vi "CRYMain.vi"() -> ()   [LabVIEW 2013]
uses:
  CRYMainGlobal.vi
  CRYProject/CRYProject Editor Global.vi
  CRYSystem/Task Sequence/CRYProject Run Control Global.vi
  CRYSystem/Data/CRYData & result stacks global.vi
  CRYCurveLibrary/Global/CRYCurve Library Global.vi
panel:
  in  "Tested:":string caption="己测:"
  in  "Curve Library":bool
  in  "OneSetup":bool
  in  "OneCalMic":bool
  in  "OneSelfTest":bool
  in  "Seq Continue":bool
  in  "Wave Lib":bool
  in  "TF Lib":bool
  in  "Value Lib":bool
  in  "SetCalibration":bool
  in  "SetSoundCard":bool
  out "Elapsed":string="00.00"
  in  "Pause":bool
  in  "S/N:":string caption="序号:"
  in  "Lot:":string caption="品名:"
  in  "Manual":bool
  in  "About":bool
  in  "Company Site":bool
  in  "RTA":bool
  in  "Spectral":bool
  in  "Oscillo":bool
  in  "MultiMeter":bool
  in  "SignalGen":bool
  in  "Document":bool
  in  "Data View":bool
  in  "Step Setup":bool
  in  "Curve Lib":bool
  in  "Project":bool
  in  "Pre Window:State":T1(ring)
  in  "DockCommand":string
  out "DockInsert":i32
  in  "Redo":bool
  in  "Continue":bool
  in  "Start":bool
  in  "AddStep":bool
  out "Seq cont border":bool
  in  "stop":bool
  in  "Calibration setup":string
  in  "Hardware setup":string
  out "no key":bool
  out "Key Val":string
  in  "Seq running":bool
  out "Verdict":bool
  out "Margin":string="0.0"
  out "Category Name":string
  in  "StateName":string
  out "State":u8(slide)=49 scale=0.0..100.0
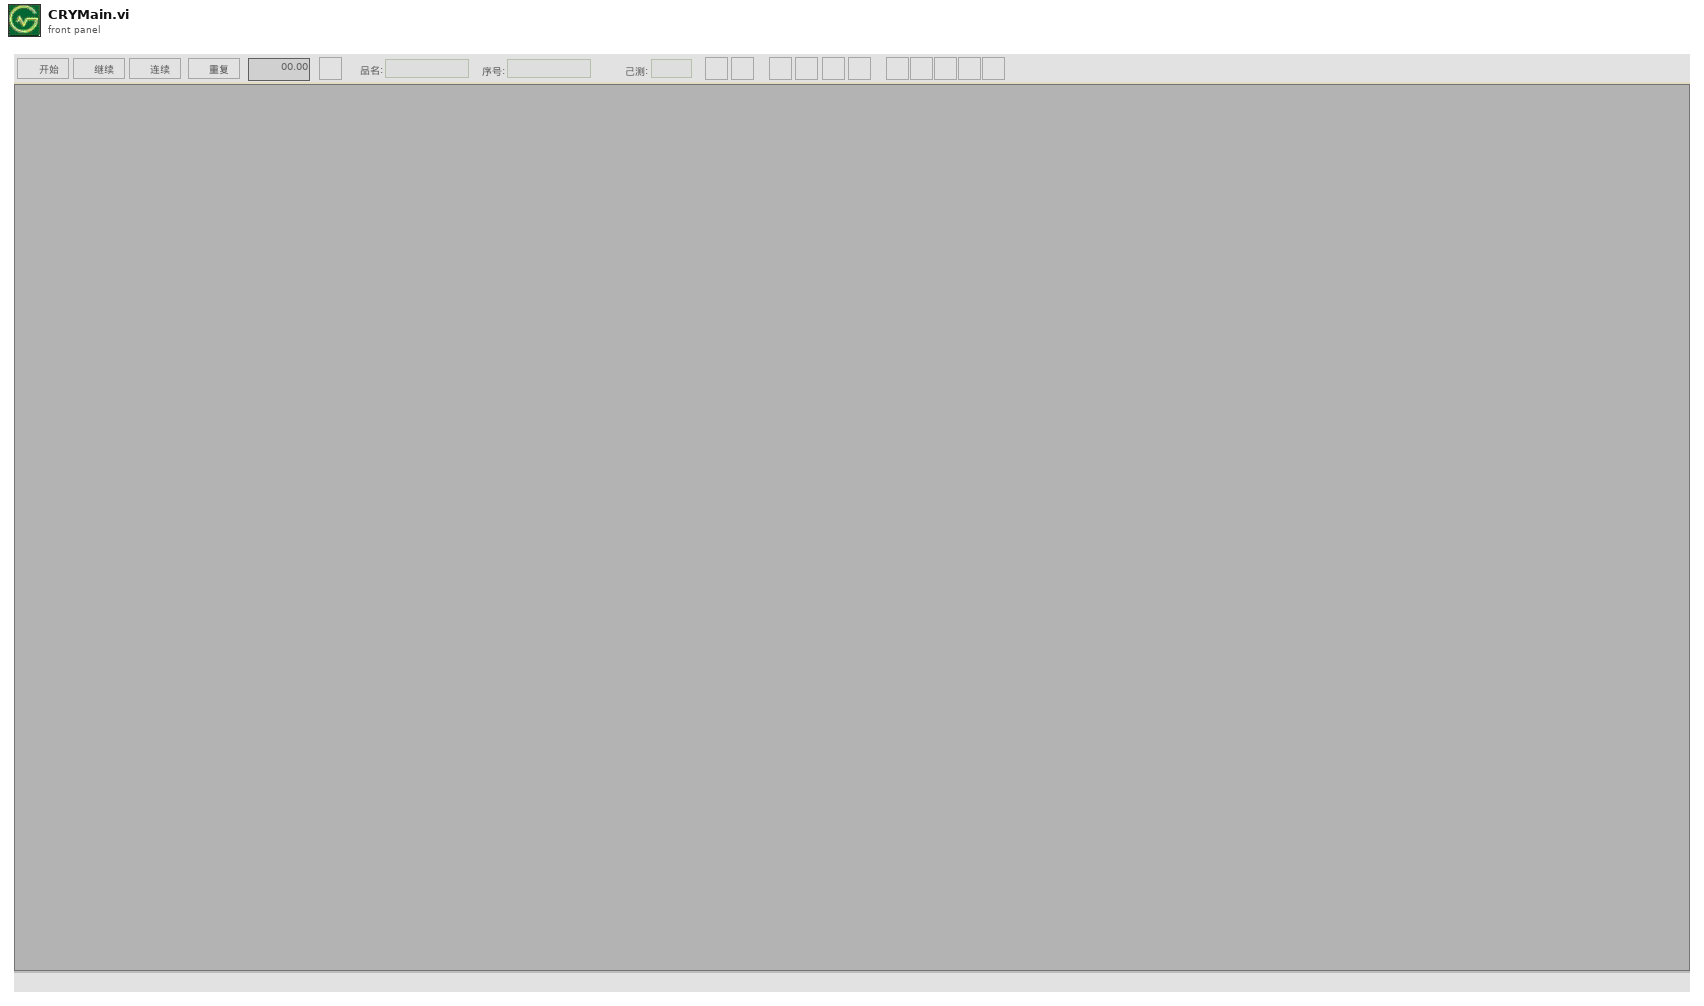
[diagram p1: front panel]
types:
  T1 = enum32{"Invalid", "Standard", "Closed", "Hidden", "Minimized", "Maximized"}
  T2 = enum32{"English", "Chinese", "Korean", "Japanese", "Russian", "Chinese traditional"}
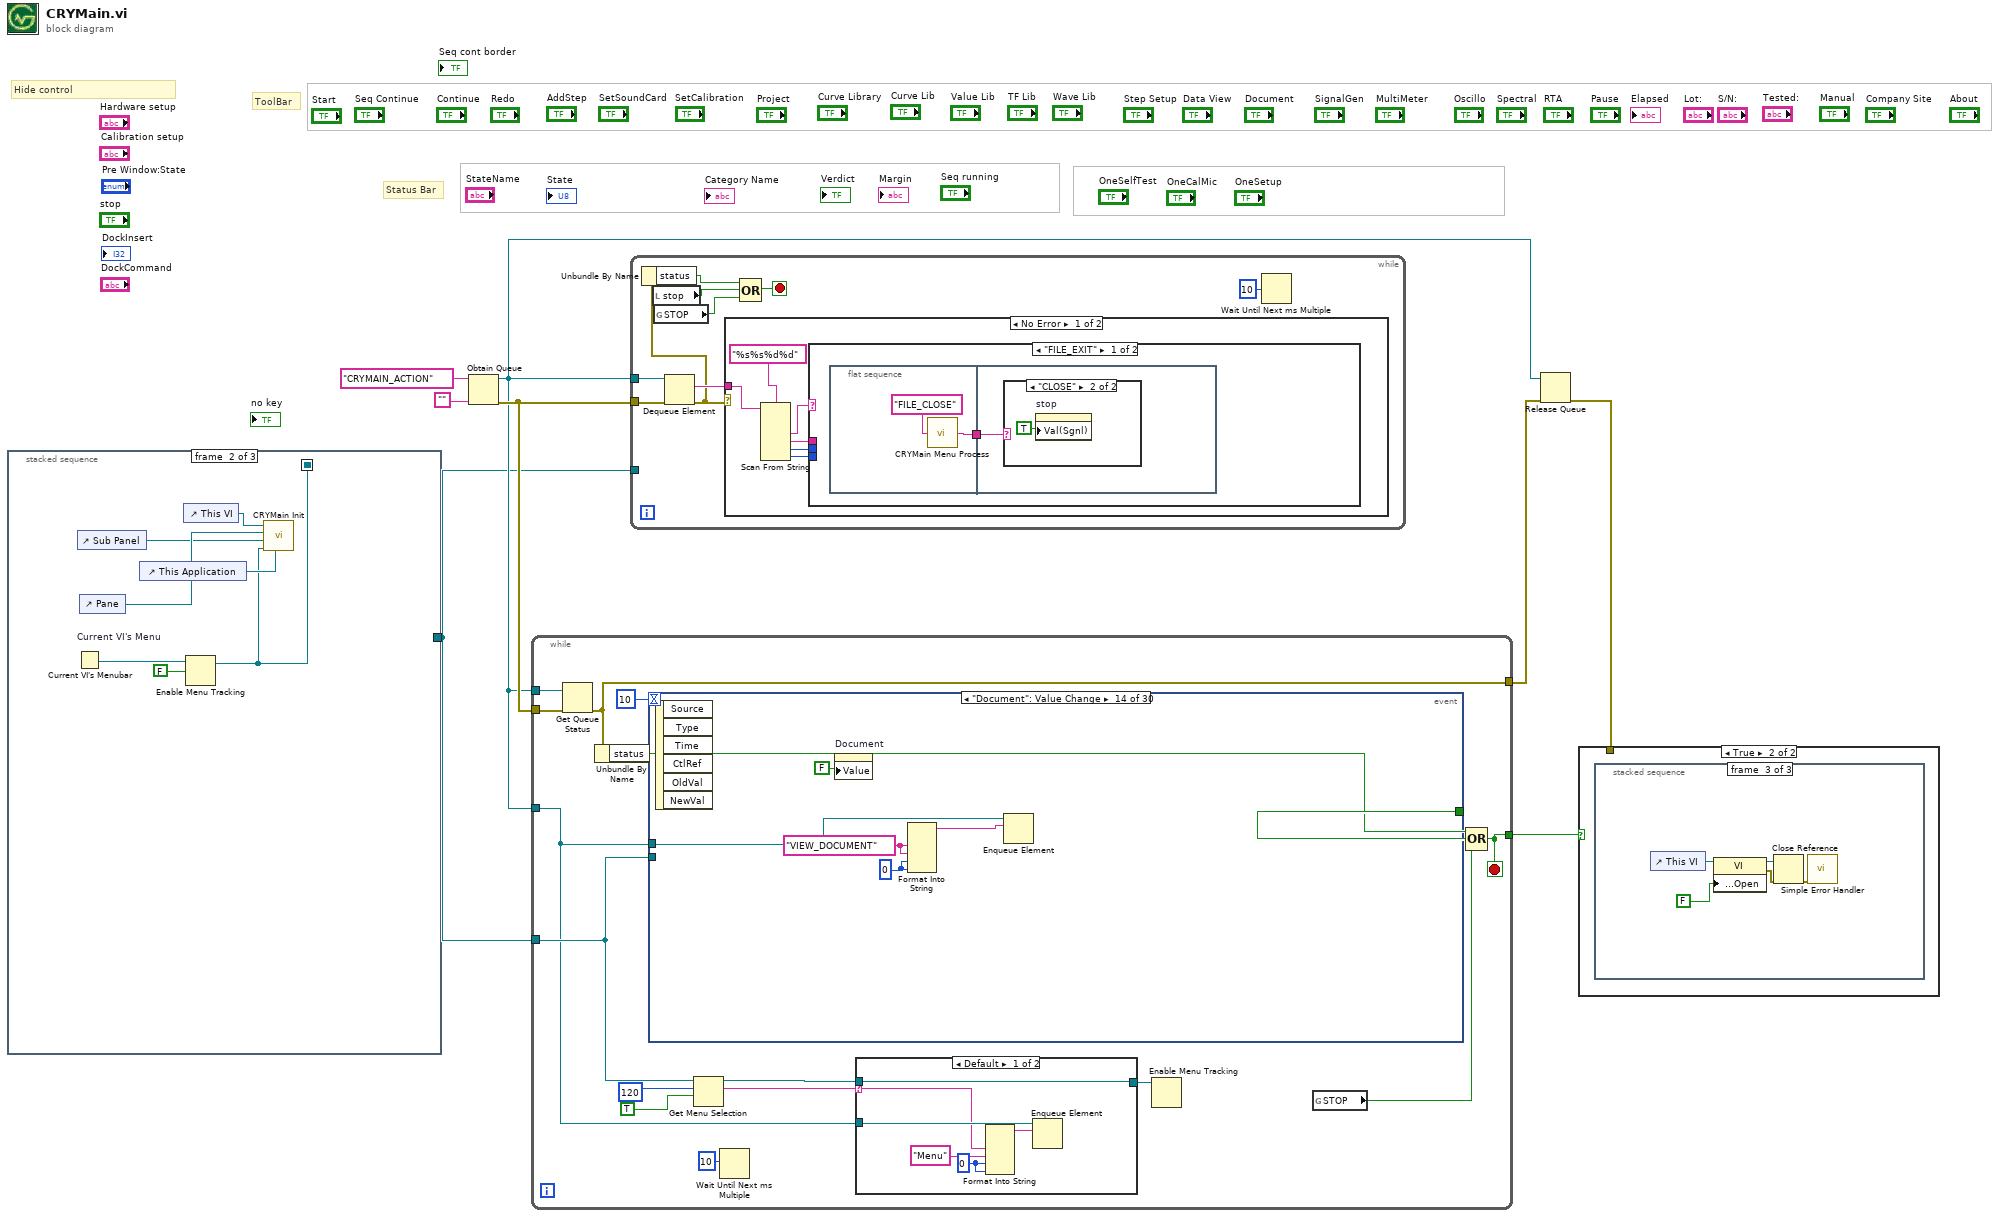
[diagram p0: block diagram]
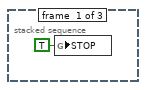
[diagram p3: hidden frame]
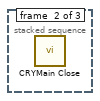
[diagram p4: hidden frame]
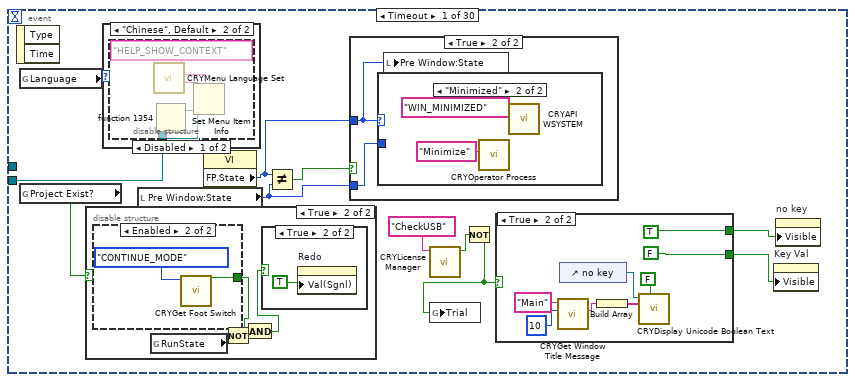
[diagram p5: hidden frame]
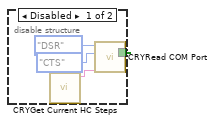
[diagram p7: hidden frame]
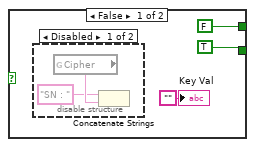
[diagram p9: hidden frame]
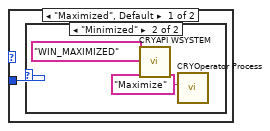
[diagram p14: hidden frame]
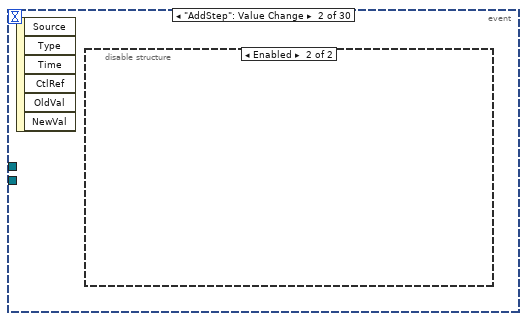
[diagram p16: hidden frame]
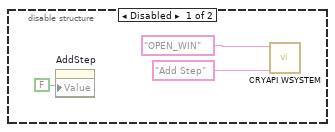
[diagram p17: hidden frame]
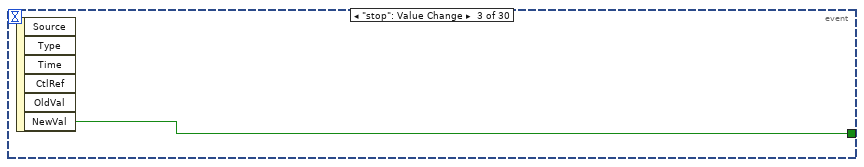
[diagram p18: hidden frame]
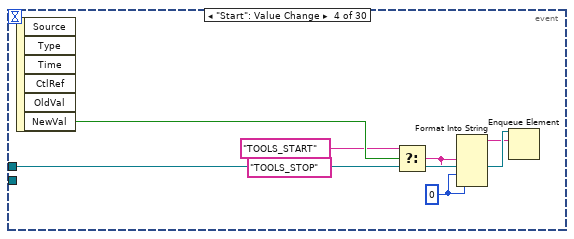
[diagram p19: hidden frame]
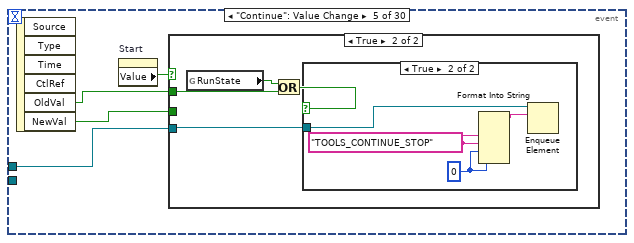
[diagram p20: hidden frame]
diagram:
  # "ToolBar"
  # "Status Bar"
  # "Hide control"
  n1 = stacked-sequence {
    seq-local: [_ w21 _] -> [_ _ w30]
    tunnel: [_ _ w29] -> w2
    frame #0 {
      n2 = global read "CRYMainGlobal.vi" "Launch Mode"() -> (w9:enum32{"CRY6181", "CRY6181 One"})
      n3 = property class="VI"() -> ("FP.State"=w15:T1)  [unwired: 2 in, 2 out]
      n4 = case shown="\"CRY6181 One\"" w9 {
        tunnel: ["CRY6181 One" ("Kind") "Main" ("Kind")] -> w13
        tunnel: [0 ("Error No") 0 ("Error No")] -> w12
        frame "CRY6181 One" {
        }
        frame "CRY6181", Default {
        }
      }
      n5 = call "CRYPreLoad StepRefs.vi"() -> ()  [unwired: 11 in, 1 out]
      n6 = local write "Pre Window:State"(w15) -> ()
      n7 = local write "Continue"(FALSE ("Continue")) -> ()
      n8 = local write "stop"(FALSE ("stop")) -> ()
      n9 = control-ref of="This VI"() -> (w11:refnum<vi>)
      n10 = call "CRYGet Window Title Message.vi"("No"=w12, "Kind"=w13) -> ("Multibyte String"=w10:string)  [unwired: 4 in, 5 out]
      n11 = property class="VI"(reference=w11, "Front Panel.Title"=w10) -> ()  [unwired: 1 in, 2 out]
    }
    frame #1 {
      n12 = Current VI's Menubar "Current VI's Menu"() -> (w24:refnum<k9>)
      n13 = control-ref of="Sub Panel"() -> (w26:refnum<vi>)
      n14 = control-ref of="Pane"() -> (w27:refnum<vi>)
      n15 = control-ref of="This Application"() -> (w22:refnum<vi>)
      n16 = control-ref of="This VI"() -> (w23:refnum<vi>)
      n17 = Enable Menu Tracking(3:FALSE ("enable (T)"), 4:w24) -> (1:w21:refnum<k9>)  [unwired: 1 in, 1 out]
      n18 = call "CRYMain Init.vi"("This Application"=w22, "Menu Refnum"=w21, "Main View SubPanel"=w26, "Pane"=w27, "Main VI Ref"=w23) -> ()  [unwired: 7 out]
    }
    frame #2 {
      w32 = FALSE ("Visible")
      n19 = invoke on="Sub Panel" class="SubPnl" method="FitControlToPane"() -> ()  [unwired: 3 in, 3 out]
      n20 = property on="DockCommand" class="Str"("Visible"=w32) -> ()  [unwired: 2 in, 2 out]
      n21 = property on="DockInsert" class="DigNum (strict)"("Visible"=w32) -> ()  [unwired: 2 in, 2 out]
      n22 = global write "CRYMainGlobal.vi" "Main Load"(TRUE ("Main Load")) -> ()
      n23 = Enable Menu Tracking(3:TRUE ("enable (T)"), 4:w30) -> (1:w29:refnum<k9>)  [unwired: 1 in, 1 out]
    }
  }
  n24 = Obtain Queue(name (unnamed)="CRYMAIN_ACTION" ("YAxisTitle"), element data type="" ("Action Type")) -> (queue out=w4:refnum<queue>, error out=w6:errorcluster)  [unwired: 3 in, 1 out]
  n25 = while {
    tunnel: w6 -> [w47]
    tunnel: w4 -> [w48]
    tunnel: [w44] -> w5
    tunnel: w2 -> [w35]
    tunnel: w4 -> [w34]
    tunnel: [w38] -> w3
    stop <- w38 stop-if-true
    n26 = Get Queue Status(queue=w48, error in (no error)=w47) -> (error out=w44:errorcluster)  [unwired: 8 out]
    n27 = Unbundle By Name(w44) -> ("status"=w45:bool)
    n28 = event shown="[13] \"Document\": Value Change" {
      selector: _ -> [_ _ _ _ _ _ _ _ _ _ _ _ _ _ _ _ _ _ _ _ _ _ _ _ _ _ _ _ _ _]
      dyn-events: _ -> [_ _ _ _ _ _ _ _ _ _ _ _ _ _ _ _ _ _ _ _ _ _ _ _ _ _ _ _ _ _]
      timeout: 10 -> [_ _ _ _ _ _ _ _ _ _ _ _ _ _ _ _ _ _ _ _ _ _ _ _ _ _ _ _ _ _]
      tunnel: [_ _ w100 _ _ _ _ _ _ _ _ _ _ _ _ _ _ _ _ _ _ _ _ _ _ _ _ _ _ FALSE ("NewVal")] -> w46
      tunnel: w34 -> [_ _ _ w107 w111 w132 w151 w154 w159 _ w168 w193 w198 w203 w208 w214 w220 w226 w232 w239 _ w251 _ w255 w261 w265 w271 w276 w281 w291]
      tunnel: w35 -> [w56 _ _ _ _ _ _ _ _ _ _ _ _ _ _ _ _ _ _ _ _ _ _ _ _ _ _ _ _ _]
      event Timeout {
        n29 = event-data() -> ()  [unwired: 3 out]
        n30 = global read "CRYMainGlobal.vi" "Language"() -> (w55:T2)
        n31 = global read "CRYProject Editor Global.vi" "Project Exist?"() -> (w49:bool)
        n32 = case shown="True" w49 {
          frame False {
          }
          frame True {
            n33 = disable-structure shown="Enabled" {
              disable-tunnel: [w64 w69] -> w62
              frame Disabled {
                n34 = call "CRYGet Current HC Steps.vi"() -> ("Hardware setup flattened Out"=w65:string)  [unwired: 10 in, 1 out]
                n35 = call "CRYRead COM Port.vi"("Hardware setup (if array not wired)"=w65, "Status Line 2"=enum16{"CTS", "DSR", "RI", "CD"}."CTS", "Status Line"=enum16{"CTS", "DSR", "RI", "CD"}."DSR") -> ("State 2 (Start & Continue)"=w64:bool)  [unwired: 6 in, 2 out]
              }
              frame Enabled {
                n36 = call "CRYGet Foot Switch.vi"("Switch Mode"=enum16{"ONESTOP_MODE", "CONTINUE_MODE"}."CONTINUE_MODE") -> ("bResult"=w69:bool)  [unwired: 10 in]
              }
            }
            n37 = global read "CRYProject Run Control Global.vi" "RunState"() -> (w63:bool)
            n38 = Not(x=w63) -> (.not. x?=w60:bool)
            n39 = And(x=w62, y=w60) -> (x .and. y?=w61:bool)
            n40 = case shown="True" w61 {
              frame False {
              }
              frame True {
                n41 = property on="Redo" class="Bool (strict)"("Val(Sgnl)"=TRUE ("Value (Signaling)")) -> ()  [unwired: 2 in, 2 out]
              }
            }
          }
        }
        n42 = case shown="\"Chinese\", Default" w55 {
          tunnel: w56 -> [_ w84]
          frame "Korean", "Chinese traditional" {
          }
          frame "Chinese", Default {
            n43 = disable-structure shown="Disabled" {
              disable-tunnel: w84 -> [w85 _]
              frame Disabled {
                n44 = call "CRYMenu Language Set.vi"("sID"="HELP_SHOW_CONTEXT" ("item tag")) -> ("sMultibyte_Out"=w88:string, "sID_Out"=w89:string)  [unwired: 7 in, 2 out]
                n45 = fn#1354() -> (1:w86:bool)  [unwired: 1 out]
                n46 = Set Menu Item Info(6:w86, 7:w89, 10:w88, 11:w85) -> ()  [unwired: 1 in, 4 out]
              }
              frame Enabled {
              }
            }
          }
        }
        n47 = local read "Pre Window:State"() -> (w57:T1)
        n48 = property class="VI"() -> ("FP.State"=w58:T1)  [unwired: 2 in, 2 out]
        n49 = Not Equal?(x=w58, y=w57) -> (x != y?=w59:bool)
        n50 = case shown="True" w59 {
          tunnel: w58 -> [_ w91]
          tunnel: w57 -> [_ w90]
          frame False {
          }
          frame True {
            n51 = case shown="\"Minimized\"" w91 {
              tunnel: w90 -> [w92 _]
              frame "Maximized", Default {
                n52 = case shown="\"Minimized\"" w92 {
                  frame "Invalid", Default {
                  }
                  frame "Minimized" {
                    n53 = call "CRYAPI WSYSTEM.vi"("sAction"="WIN_MAXIMIZED") -> ()  [unwired: 7 in, 4 out]
                    n54 = call "CRYOperator Process.vi"("sAction"="Maximize") -> ()  [unwired: 10 in, 1 out]
                  }
                }
              }
              frame "Minimized" {
                n55 = call "CRYOperator Process.vi"("sAction"="Minimize") -> ()  [unwired: 10 in, 1 out]
                n56 = call "CRYAPI WSYSTEM.vi"("sAction"="WIN_MINIMIZED") -> ()  [unwired: 7 in, 4 out]
              }
            }
            n57 = local write "Pre Window:State"(w91) -> ()
          }
        }
        n58 = call "CRYLicense Manager.vi"("sAction"="CheckUSB") -> ("Test Result"=w51:bool)  [unwired: 9 in, 1 out]
        n59 = Not(x=w51) -> (.not. x?=w50:bool)
        n60 = global write "CRYMainGlobal.vi" "Trial"(w50) -> ()
        n61 = case shown="True" w50 {
          tunnel: [FALSE ("Visible") TRUE ("Visible")] -> w53
          tunnel: [TRUE ("Visible") FALSE ("Visible")] -> w54
          frame False {
            n62 = disable-structure shown="Disabled" {
              frame Disabled {
                n63 = global read "CRYMainGlobal.vi" "Cipher"() -> (w75:string)
                n64 = Concatenate Strings("SN : " ("string"), w75) -> ()  [unwired: 1 out]
              }
              frame Enabled {
              }
            }
            "Key Val" <- "" ("Key Val")
          }
          frame True {
            n65 = call "CRYGet Window Title Message.vi"("No"=10, "Kind"="Main") -> ("Unicode String"=w76:string)  [unwired: 4 in, 5 out]
            n66 = control-ref of="no key"() -> (w81:refnum<vi>)
            n67 = Build Array(w76) -> (w80:string[])
            n68 = call "CRYDisplay Unicode Boolean Text.vi"("Interpret as Unicode (T)"=FALSE, "Boolean Texts [4]"=w80, "Boolean Reference"=w81) -> ()  [unwired: 5 in, 2 out]
          }
        }
        n69 = property on="Key Val" class="Str"("Visible"=w54) -> ()  [unwired: 2 in, 2 out]
        n70 = property on="no key" class="Bool (strict)"("Visible"=w53) -> ()  [unwired: 2 in, 2 out]
      }
      event "AddStep": Value Change {
        n71 = event-data() -> ()  [unwired: 7 out]
        n72 = disable-structure shown="Enabled" {
          frame Disabled {
            n73 = property on="AddStep" class="Bool (strict)"("Value"=FALSE ("AddStep")) -> ()  [unwired: 2 in, 2 out]
            n74 = call "CRYAPI WSYSTEM.vi"("sData"="Add Step", "sAction"="OPEN_WIN") -> ()  [unwired: 2 in, 8 out]
          }
          frame Enabled {
          }
        }
      }
      event "stop": Value Change {
        n75 = event-data() -> ("NewVal"=w100:bool)  [unwired: 6 out]
      }
      event "Start": Value Change {
        w101 = 0 ("input 3")
        n76 = event-data() -> ("NewVal"=w106:bool)  [unwired: 6 out]
        n77 = Select(t="TOOLS_START" ("input 1"), s=w106, f="TOOLS_STOP" ("input 1")) -> (s? t:f=w102:string)
        n78 = Format Into String(w102, w102, w101, w101) -> (resulting string=w105:string)  [unwired: 3 in, 1 out]
        n79 = Enqueue Element(queue=w107, element=w105) -> ()  [unwired: 1 in, 4 out]
      }
      event "Continue": Value Change {
        n80 = event-data() -> ("OldVal"=w108:bool, "NewVal"=w110:bool)  [unwired: 5 out]
        n81 = property on="Start" class="Bool (strict)"() -> ("Value"=w109:bool)  [unwired: 2 in, 2 out]
        n82 = case shown="True" w109 {
          tunnel: w111 -> [w119 w120]
          tunnel: w110 -> [w118 _]
          tunnel: w108 -> [_ w121]
          frame False {
            n83 = Select(t="TOOLS_CONTINUE" ("input 1"), s=w118, f="TOOLS_CONTINUE_STOP" ("input 1")) -> (s? t:f=w112:string)
            n84 = Format Into String(w112, w112, 0 ("input 2"), 0 ("input 3")) -> (resulting string=w116:string)  [unwired: 3 in, 1 out]
            n85 = Enqueue Element(queue=w119, element=w116) -> ()  [unwired: 1 in, 4 out]
          }
          frame True {
            n86 = global read "CRYProject Run Control Global.vi" "RunState"() -> (w123:bool)
            n87 = Or(x=w123, y=w121) -> (x .or. y?=w122:bool)
            n88 = case shown="True" w122 {
              tunnel: w120 -> [_ w125]
              frame False {
                n89 = property on="Continue" class="Bool (strict)"("Value"=FALSE ("Continue")) -> ()  [unwired: 2 in, 2 out]
              }
              frame True {
                w126 = 0 ("input 3")
                w128 = "TOOLS_CONTINUE_STOP" ("input 1")
                n90 = Format Into String(w128, w128, w126, w126) -> (resulting string=w127:string)  [unwired: 3 in, 1 out]
                n91 = Enqueue Element(queue=w125, element=w127) -> ()  [unwired: 1 in, 4 out]
              }
            }
          }
        }
      }
      event "Redo": Value Change {
        n92 = event-data() -> ("OldVal"=w129:bool, "NewVal"=w131:bool)  [unwired: 5 out]
        n93 = property on="Start" class="Bool (strict)"() -> ("Value"=w130:bool)  [unwired: 2 in, 2 out]
        n94 = case shown="True" w130 {
          tunnel: w132 -> [w139 w143]
          tunnel: w131 -> [w138 _]
          tunnel: w129 -> [_ w141]
          frame False {
            w134 = 0 ("input 3")
            n95 = Select(t="TOOLS_REDO" ("input 1"), s=w138, f="TOOLS_STOP" ("input 1")) -> (s? t:f=w133:string)
            n96 = Format Into String(w133, w133, w134, w134) -> (resulting string=w135:string)  [unwired: 3 in, 1 out]
            n97 = Enqueue Element(queue=w139, element=w135) -> ()  [unwired: 1 in, 4 out]
          }
          frame True {
            n98 = global read "CRYProject Run Control Global.vi" "RunState"() -> (w142:bool)
            n99 = Or(x=w142, y=w141) -> (x .or. y?=w140:bool)
            n100 = case shown="True" w140 {
              tunnel: w143 -> [_ w145]
              frame False {
                n101 = property on="Redo" class="Bool (strict)"("Value"=FALSE ("Redo")) -> ()  [unwired: 2 in, 2 out]
              }
              frame True {
                w146 = 0 ("input 3")
                w148 = "TOOLS_STOP" ("input 1")
                n102 = Format Into String(w148, w148, w146, w146) -> (resulting string=w147:string)  [unwired: 3 in, 1 out]
                n103 = Enqueue Element(queue=w145, element=w147) -> ()  [unwired: 1 in, 4 out]
              }
            }
          }
        }
      }
      event "Project": Value Change {
        w150 = "VIEW_PROJECT" ("input 1")
        w152 = 0 ("input 3")
        n104 = event-data() -> ()  [unwired: 7 out]
        n105 = property on="Project" class="Bool (strict)"("Value"=FALSE ("Project")) -> ()  [unwired: 2 in, 2 out]
        n106 = Format Into String(w150, w150, w152, w152) -> (resulting string=w153:string)  [unwired: 3 in, 1 out]
        n107 = Enqueue Element(queue=w151, element=w153) -> ()  [unwired: 1 in, 4 out]
      }
      event "SetSoundCard": Value Change {
        w155 = "VIEW_SOUNDCARD" ("input 1")
        w156 = 0 ("input 3")
        n108 = event-data() -> ()  [unwired: 7 out]
        n109 = property on="SetSoundCard" class="Bool (strict)"("Value"=FALSE ("Project")) -> ()  [unwired: 2 in, 2 out]
        n110 = Format Into String(w155, w155, w156, w156) -> (resulting string=w157:string)  [unwired: 3 in, 1 out]
        n111 = Enqueue Element(queue=w154, element=w157) -> ()  [unwired: 1 in, 4 out]
      }
      event "SetCalibration": Value Change {
        w160 = "VIEW_CALIBRATION" ("input 1")
        w161 = 0 ("input 3")
        n112 = event-data() -> ()  [unwired: 7 out]
        n113 = property on="SetCalibration" class="Bool (strict)"("Value"=FALSE ("Project")) -> ()  [unwired: 2 in, 2 out]
        n114 = Format Into String(w160, w160, w161, w161) -> (resulting string=w162:string)  [unwired: 3 in, 1 out]
        n115 = Enqueue Element(queue=w159, element=w162) -> ()  [unwired: 1 in, 4 out]
      }
      event "Seq Continue": Value Change {
        n116 = event-data() -> ("NewVal"=w164:bool)  [unwired: 6 out]
        n117 = global read "CRYMainGlobal.vi" "Seq Continue Ref"() -> (w165:refnum<vi>)
        n118 = property class="Bool (strict)"(reference=w165, "Val(Sgnl)"=w164) -> ()  [unwired: 1 in, 2 out]
      }
      event "Curve Lib", "Value Lib", "TF Lib", "Wave Lib", "Curve Library": Value Change {
        n119 = event-data() -> ("CtlRef"=w167:refnum<vi>)  [unwired: 6 out]
        n120 = disable-structure shown="Disabled" {
          disable-tunnel: w167 -> [w178 _]
          frame Disabled {
            n121 = property class="Bool (strict)"(reference=w178, "Value"=FALSE ("Project")) -> (reference out=w176:refnum<vi>, error out=w175:errorcluster)  [unwired: 1 in]
            n122 = property class="Bool (strict)"(reference=w176, error in=w175) -> ("Label.Text"=w174:string)  [unwired: 2 out]
            n123 = case shown="Default" w174 {
              tunnel: ["Curves" "Values" "Results" "WFM"] -> w173
              frame "Curve Lib" {
              }
              frame "Value Lib" {
              }
              frame "TF Lib" {
              }
              frame Default {
              }
            }
            n124 = global read "CRYCurve Library Global.vi" "Curve Library Tab"() -> (w170:refnum<vi>)
            n125 = flat-sequence {
              tunnel: w173 -> [w179]
              frame #0 {
                n126 = global write "CRYCurve Library Global.vi" "CurLib Type"(w179) -> ()
              }
              frame #1 {
                n127 = call "CRYSet Title Name and Icon from Type.vi"() -> ()  [unwired: 12 in]
              }
            }
            n128 = case shown="\"False\", Default" w174 {
              tunnel: [u32 3 ("Curve Lib Tab Index") u32 0 ("Curve Lib Tab Index") u32 1 ("Curve Lib Tab Index") u32 2 ("Curve Lib Tab Index")] -> w171
              frame "False", Default {
              }
              frame "Curve Lib" {
              }
              frame "Value Lib" {
              }
              frame "TF Lib" {
              }
            }
            n129 = To Variant(anything=w171) -> (Variant=w172:variant)
            n130 = property class="TabCtl"(reference=w170, "Value"=w172) -> (reference out=w169:refnum<vi>)  [unwired: 1 in, 1 out]
            n131 = flat-sequence {
              tunnel: w169 -> [_]
              frame #0 {
                n132 = call "CRYUpdate Buttons.vi"() -> ()  [unwired: 1 in, 11 out]
              }
            }
          }
          frame Enabled {
          }
        }
        n133 = property on="Curve Library" class="Bool (strict)"("Value"=FALSE ("Curve Library")) -> ()  [unwired: 2 in, 2 out]
        n134 = flat-sequence {
          tunnel: w168 -> [w188]
          frame #0 {
            w189 = "VIEW_CURVES_LIBRARY" ("input 1")
            w190 = 0 ("input 3")
            n135 = Format Into String(w189, w189, w190, w190) -> (resulting string=w191:string)  [unwired: 3 in, 1 out]
            n136 = Enqueue Element(queue=w188, element=w191) -> ()  [unwired: 1 in, 4 out]
          }
        }
      }
      event "Step Setup": Value Change {
        w194 = "VIEW_STEP_SETUP" ("input 1")
        w195 = 0 ("input 3")
        n137 = event-data() -> ()  [unwired: 7 out]
        n138 = property on="Step Setup" class="Bool (strict)"("Value"=FALSE ("Project")) -> ()  [unwired: 2 in, 2 out]
        n139 = Format Into String(w194, w194, w195, w195) -> (resulting string=w196:string)  [unwired: 3 in, 1 out]
        n140 = Enqueue Element(queue=w193, element=w196) -> ()  [unwired: 1 in, 4 out]
      }
      event "Data View": Value Change {
        w199 = "VIEW_DATA_VIEW" ("input 1")
        w200 = 0 ("input 3")
        n141 = event-data() -> ()  [unwired: 7 out]
        n142 = property on="Data View" class="Bool (strict)"("Value"=FALSE ("Project")) -> ()  [unwired: 2 in, 2 out]
        n143 = Format Into String(w199, w199, w200, w200) -> (resulting string=w201:string)  [unwired: 3 in, 1 out]
        n144 = Enqueue Element(queue=w198, element=w201) -> ()  [unwired: 1 in, 4 out]
      }
      event "Document": Value Change {
        w204 = "VIEW_DOCUMENT" ("input 1")
        w205 = 0 ("input 3")
        n145 = event-data() -> ()  [unwired: 7 out]
        n146 = property on="Document" class="Bool (strict)"("Value"=FALSE ("Project")) -> ()  [unwired: 2 in, 2 out]
        n147 = Format Into String(w204, w204, w205, w205) -> (resulting string=w206:string)  [unwired: 3 in, 1 out]
        n148 = Enqueue Element(queue=w203, element=w206) -> ()  [unwired: 1 in, 4 out]
      }
      event "SignalGen": Value Change {
        w209 = 0 ("input 2")
        n149 = event-data() -> ()  [unwired: 7 out]
        n150 = property on="SignalGen" class="Bool (strict)"("Value"=FALSE ("MultiMeter")) -> ()  [unwired: 2 in, 2 out]
        n151 = Format Into String("OPERATOR_SIGGEN" ("input 1"), "Menu" ("input 1"), w209, w209) -> (resulting string=w211:string)  [unwired: 3 in, 1 out]
        n152 = Enqueue Element(queue=w208, element=w211) -> ()  [unwired: 1 in, 4 out]
      }
      event "MultiMeter": Value Change {
        w215 = 0 ("input 2")
        n153 = event-data() -> ()  [unwired: 7 out]
        n154 = property on="MultiMeter" class="Bool (strict)"("Value"=FALSE ("MultiMeter")) -> ()  [unwired: 2 in, 2 out]
        n155 = Format Into String("OPERATOR_MULTIMETER" ("input 1"), "Menu" ("input 1"), w215, w215) -> (resulting string=w217:string)  [unwired: 3 in, 1 out]
        n156 = Enqueue Element(queue=w214, element=w217) -> ()  [unwired: 1 in, 4 out]
      }
      event "Oscillo": Value Change {
        w221 = 0 ("input 2")
        n157 = event-data() -> ()  [unwired: 7 out]
        n158 = property on="Oscillo" class="Bool (strict)"("Value"=FALSE ("Oscillo")) -> ()  [unwired: 2 in, 2 out]
        n159 = Format Into String("OPERATOR_OSCILLOSCOPE" ("input 1"), "Menu" ("input 1"), w221, w221) -> (resulting string=w223:string)  [unwired: 3 in, 1 out]
        n160 = Enqueue Element(queue=w220, element=w223) -> ()  [unwired: 1 in, 4 out]
      }
      event "Spectral": Value Change {
        w227 = 0 ("input 2")
        n161 = event-data() -> ()  [unwired: 7 out]
        n162 = property on="Spectral" class="Bool (strict)"("Value"=FALSE ("Spectral")) -> ()  [unwired: 2 in, 2 out]
        n163 = Format Into String("OPERATOR_SPECTRUM" ("input 1"), "Menu" ("input 1"), w227, w227) -> (resulting string=w229:string)  [unwired: 3 in, 1 out]
        n164 = Enqueue Element(queue=w226, element=w229) -> ()  [unwired: 1 in, 4 out]
      }
      event "RTA": Value Change {
        w233 = 0 ("input 2")
        n165 = event-data() -> ()  [unwired: 7 out]
        n166 = property on="RTA" class="Bool (strict)"("Value"=FALSE ("RTA")) -> ()  [unwired: 2 in, 2 out]
        n167 = Format Into String("OPERATOR_RTA" ("input 1"), "Menu" ("input 1"), w233, w233) -> (resulting string=w235:string)  [unwired: 3 in, 1 out]
        n168 = Enqueue Element(queue=w232, element=w235) -> ()  [unwired: 1 in, 4 out]
      }
      event "Pause": Value Change {
        n169 = event-data() -> ("NewVal"=w238:bool)  [unwired: 6 out]
        n170 = flat-sequence {
          tunnel: w238 -> [w240]
          tunnel: w239 -> [w241]
          tunnel: [w241] -> w237
          tunnel: w237 -> [w242]
          frame #0 {
            n171 = global write "CRYData & result stacks global.vi" "Pause"(w240) -> ()
          }
          frame #1 {
            w243 = 0 ("input 2")
            n172 = Format Into String("TOOLS_LOTPAUSE" ("input 1"), "Menu" ("input 1"), w243, w243) -> (resulting string=w245:string)  [unwired: 3 in, 1 out]
            n173 = Enqueue Element(queue=w242, element=w245) -> ()  [unwired: 1 in, 4 out]
          }
        }
      }
      event "Lot:": Value Change {
        n174 = event-data() -> ("NewVal"=w247:string)  [unwired: 6 out]
        n175 = global write "CRYData & result stacks global.vi" "Lot #"(w247) -> ()
      }
      event "DockInsert": Value Change {
        n176 = event-data() -> ("NewVal"=w249:i32)  [unwired: 6 out]
        n177 = local read "DockCommand"() -> (w250:string)
        n178 = Format Into String(w250, "Dock_Insert" ("input 2"), w249, 0 ("input 3")) -> (resulting string=w253:string)  [unwired: 3 in, 1 out]
        n179 = Enqueue Element At Opposite End(queue=w251, element=w253) -> ()  [unwired: 1 in, 4 out]
      }
      event "S/N:": Value Change {
        n180 = event-data() -> ("NewVal"=w254:string)  [unwired: 6 out]
        n181 = global write "CRYData & result stacks global.vi" "Serial #"(w254) -> ()
      }
      event "Manual": Value Change {
        w257 = "HELP_USER_MANUAL" ("input 1")
        w258 = 0 ("input 3")
        n182 = event-data() -> ()  [unwired: 7 out]
        n183 = property on="Manual" class="Bool (strict)"("Value"=FALSE ("RTA")) -> ()  [unwired: 2 in, 2 out]
        n184 = Format Into String(w257, w257, w258, w258) -> (resulting string=w259:string)  [unwired: 3 in, 1 out]
        n185 = Enqueue Element(queue=w255, element=w259) -> ()  [unwired: 1 in, 4 out]
      }
      event "Company Site": Value Change {
        w262 = "HELP_COMPANYWEB" ("input 1")
        w263 = 0 ("input 3")
        n186 = event-data() -> ()  [unwired: 7 out]
        n187 = property on="Company Site" class="Bool (strict)"("Value"=FALSE ("RTA")) -> ()  [unwired: 2 in, 2 out]
        n188 = Format Into String(w262, w262, w263, w263) -> (resulting string=w264:string)  [unwired: 3 in, 1 out]
        n189 = Enqueue Element(queue=w261, element=w264) -> ()  [unwired: 1 in, 4 out]
      }
      event "About": Value Change {
        w267 = "HELP_ABOUT" ("input 1")
        w268 = 0 ("input 3")
        n190 = event-data() -> ()  [unwired: 7 out]
        n191 = property on="About" class="Bool (strict)"("Value"=FALSE ("RTA")) -> ()  [unwired: 2 in, 2 out]
        n192 = Format Into String(w267, w267, w268, w268) -> (resulting string=w269:string)  [unwired: 3 in, 1 out]
        n193 = Enqueue Element(queue=w265, element=w269) -> ()  [unwired: 1 in, 4 out]
      }
      event "OneSelfTest": Value Change {
        w274 = "ONE_SELFTEST" ("input 1")
        w273 = 0 ("input 3")
        n194 = event-data() -> ()  [unwired: 7 out]
        n195 = Format Into String(w274, w274, w273, w273) -> (resulting string=w272:string)  [unwired: 3 in, 1 out]
        n196 = property on="OneSelfTest" class="Bool (strict)"("Value"=FALSE ("RTA")) -> ()  [unwired: 2 in, 2 out]
        n197 = Enqueue Element(queue=w271, element=w272) -> ()  [unwired: 1 in, 4 out]
      }
      event "OneCalMic": Value Change {
        w279 = "ONE_CALMIC" ("input 1")
        w278 = 0 ("input 3")
        n198 = event-data() -> ()  [unwired: 7 out]
        n199 = Format Into String(w279, w279, w278, w278) -> (resulting string=w277:string)  [unwired: 3 in, 1 out]
        n200 = property on="OneCalMic" class="Bool (strict)"("Value"=FALSE ("RTA")) -> ()  [unwired: 2 in, 2 out]
        n201 = Enqueue Element(queue=w276, element=w277) -> ()  [unwired: 1 in, 4 out]
      }
      event "OneSetup": Value Change {
        w284 = "ONE_SETUP" ("input 1")
        w283 = 0 ("input 3")
        n202 = event-data() -> ()  [unwired: 7 out]
        n203 = Format Into String(w284, w284, w283, w283) -> (resulting string=w282:string)  [unwired: 3 in, 1 out]
        n204 = property on="OneSetup" class="Bool (strict)"("Value"=FALSE ("RTA")) -> ()  [unwired: 2 in, 2 out]
        n205 = Enqueue Element(queue=w281, element=w282) -> ()  [unwired: 1 in, 4 out]
      }
      event Panel Close? {
        n206 = event-data() -> ()  [unwired: 5 out]
        n207 = Format Into String("FILE_EXIT" ("input 1"), "FILE_EXIT" ("input 1"), 0 ("input 2"), 0 ("input 3")) -> (resulting string=w289:string)  [unwired: 3 in, 1 out]
        n208 = Enqueue Element(queue=w291, element=w289) -> ()  [unwired: 1 in, 4 out]
        n209 = event-data("Discard?"=TRUE) -> ()  [unwired: 1 in, 1 out]
      }
    }
    n210 = Get Menu Selection(0:w35, 1:120 ("ms timeout (200)"), 2:TRUE ("block menu (F)")) -> (5:w42:refnum<k9>, 6:w39:string)  [unwired: 1 in, 3 out]
    n211 = Wait Until Next ms Multiple(millisecond multiple=u32 10 ("milliseconds to wait")) -> ()  [unwired: 1 out]
    n212 = case shown="Default" w39 {
      selector: w39 -> [w293 _]
      tunnel: w42 -> [w298 w299]
      tunnel: [w298 w299] -> w43
      tunnel: w34 -> [w296 _]
      frame Default {
        w294 = 0 ("input 2")
        n213 = Format Into String(w293, "Menu" ("input 1"), w294, w294) -> (resulting string=w297:string)  [unwired: 3 in, 1 out]
        n214 = Enqueue Element(queue=w296, element=w297) -> ()  [unwired: 1 in, 4 out]
      }
      frame "" {
      }
    }
    n215 = Enable Menu Tracking(4:w43) -> ()  [unwired: 1 in, 3 out]
    n216 = global read "CRYMainGlobal.vi" "STOP"() -> (w36:bool)
    n217 = Compound Arithmetic op=OR(w45, w46, w36) -> (w38:bool)
  }
  n218 = while {
    tunnel: w4 -> [w308]
    tunnel: w6 -> [w307]
    tunnel: w2 -> [_]
    stop <- w302 stop-if-true
    n219 = local read "stop"() -> (w306:bool)
    n220 = global read "CRYMainGlobal.vi" "STOP"() -> (w305:bool)
    n221 = Dequeue Element(queue=w308, error in (no error)=w307) -> (element=w303:string, error out=w301:errorcluster)  [unwired: 3 out]
    n222 = Unbundle By Name(w301) -> ("status"=w304:bool)
    n223 = case shown="No Error" w301 {
      tunnel: w303 -> [w309 _]
      frame No Error {
        n224 = Scan From String(format string="%s%s%d%d", input string=w309) -> (output 1=w314:string, output 2=w310:string, output 3=w311:i32, output 4=w312:i32)  [unwired: 2 in, 7 out]
        n225 = case shown="\"FILE_EXIT\"" w314 {
          selector: w314 -> [_ w321]
          tunnel: w311 -> [_ w322]
          tunnel: w312 -> [_ _]
          tunnel: w310 -> [_ w320]
          frame "FILE_EXIT" {
            n226 = flat-sequence {
              tunnel: [w317] -> w315
              tunnel: w315 -> [w318]
              frame #0 {
                n227 = call "CRYMain Menu Process.vi"("Menu String"="FILE_CLOSE") -> ("sData_Out"=w317:string)  [unwired: 4 in]
              }
              frame #1 {
                n228 = case shown="\"CLOSE\"" w318 {
                  frame "False", Default {
                  }
                  frame "CLOSE" {
                    n229 = property on="stop" class="Bool (strict)"("Val(Sgnl)"=TRUE ("Value (Signaling)")) -> ()  [unwired: 2 in, 2 out]
                  }
                }
              }
            }
          }
          frame Default {
            n230 = call "CRYMain Menu Process.vi"("Sub Menu String"=w320, "Menu String"=w321, "nData"=w322) -> ()  [unwired: 2 in, 1 out]
          }
        }
      }
      frame Error {
      }
    }
    n231 = Compound Arithmetic op=OR(w304, w306, w305) -> (w302:bool)
    n232 = Wait Until Next ms Multiple(millisecond multiple=u32 10 ("milliseconds to wait")) -> ()  [unwired: 1 out]
  }
  n233 = Release Queue(queue=w4, error in (no error)=w5) -> (error out=w1:errorcluster)  [unwired: 3 out]
  n234 = case shown="True" w3 {
    tunnel: w1 -> [_ _]
    frame False {
    }
    frame True {
      n235 = stacked-sequence {
        frame #0 {
          n236 = global write "CRYMainGlobal.vi" "STOP"(TRUE ("STOP")) -> ()
        }
        frame #1 {
          n237 = call "CRYMain Close.vi"() -> ()  [unwired: 1 out]
        }
        frame #2 {
          n238 = control-ref of="This VI"() -> (w327:refnum<vi>)
          n239 = property class="VI"(reference=w327, "Front Panel Window:Open"=FALSE ("Front Panel.Open")) -> (reference out=w328:refnum<vi>, error out=w325:errorcluster)  [unwired: 1 in]
          n240 = Close Reference(reference=w328, error in (no error)=w325) -> (error out=w324:errorcluster)
          n241 = call <vilib>:"Simple Error Handler.vi"("error in (no error)"=w324) -> ()  [unwired: 2 in, 7 out]
        }
      }
    }
  }
